vi "Stepper motor B.vi"(6 "Microstep size":T1(ring), 7 "Speed":u32=5, 8 "error in (no error)":errorcluster, 9 "Direction (A/DIO5 (Pin 21))":bool, 10 "Step (A/DIO4 (Pin 19))":bool, 11 "Enable (A/DIO0 (Pin 11))":bool) -> (0 "error out":errorcluster, 2 "Direction":bool)   [LabVIEW 2015]
uses:
  <vilib>/myRIO/Instrument Drivers/Onboard IO/DIO/DIO.lvlib
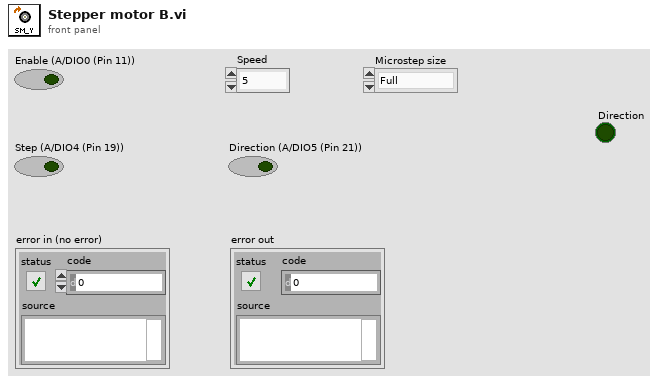
[diagram p1: front panel]
types:
  T1 = enum16{"Full", "Half", "Quarter", "Eighth", "Sixteenth"}
  T2 = cluster{"MS1 (A/DIO1 (Pin 13))":bool, "MS2 (A/DIO2 (Pin 15))":bool, "MS3 (A/DIO3 (Pin 17))":bool}
  T3 = typedef "DIO.lvlib/DIO Reference.ctl" = cluster{"myRIO Reference":T4, "DIO Channels List":T8}
  T4 = typedef "myRIO Generic Hardware Reference.ctl" = cluster{"myRIO Model":T5, "myRIO Hardware Reference":T6}
  T5 = typedef "Hardware Version Enum.ctl" = enum16{"Unknown", "myRIO-1900", "myRIO-1950", "roboRIO", "NI ELVIS RIO CM"}
  T6 = typedef "myRIO v1.0 Reference.ctl" = cluster{"Generic FPGA Reference":T7, "Allow multiple opens":bool}
  T7 = typedef "Generic FPGA Reference.ctl" = refnum<k20>
  T8 = typedef "DIO Channels List.ctl" = T9[]
  T9 = typedef "DIO Channels Enum.ctl" = enum16{"Not Connected", "C/DIO0", "C/DIO1", "C/DIO2", "C/DIO3", "C/DIO4", "C/DIO5", "C/DIO6", "C/DIO7", "A/DIO0", "A/DIO1", "A/DIO2", "A/DIO3", "A/DIO4", "A/DIO5", "A/DIO6", "A/DIO7", "A/DIO8", "A/DIO9", "A/DIO10", "A/DIO11", "A/DIO12", "A/DIO13", "A/DIO14", "A/DIO15", "B/DIO0", "B/DIO1", "B/DIO2", "B/DIO3", "B/DIO4", "B/DIO5", "B/DIO6", "B/DIO7", "B/DIO8", "B/DIO9", "B/DIO10", "B/DIO11", "B/DIO12", "B/DIO13", "B/DIO14", "B/DIO15", "LED0", "LED1", "LED2", "LED3", "Button0", "DIO/DIO0", "DIO/DIO1", "DIO/DIO2", "DIO/DIO3", "DIO/DIO4", "DIO/DIO5", "DIO/DIO6", "DIO/DIO7", "DIO/DIO8", "DIO/DIO9", "SPI/CS0", "SPI/CS1", "SPI/CS2", "SPI/CS3", "LED RADIO (Green)", "LED RADIO (Red)", "LED COMM (Green)", "LED COMM (Red)", "LED MODE (Green)", "LED MODE (Red)"}
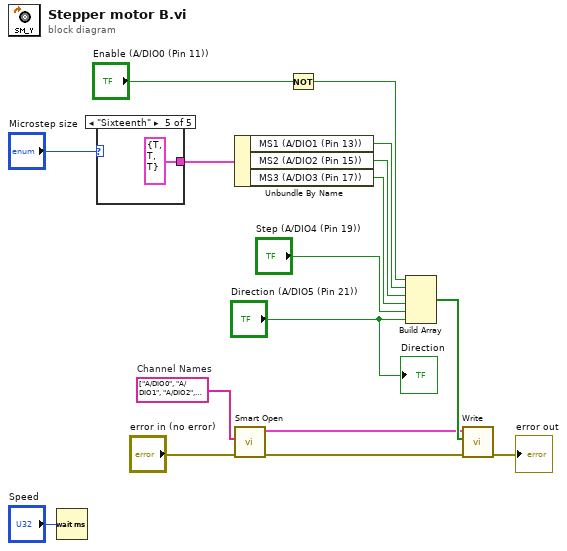
[diagram p0: block diagram]
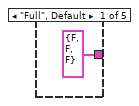
[diagram p2: hidden frame]
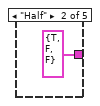
[diagram p3: hidden frame]
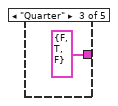
[diagram p4: hidden frame]
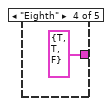
[diagram p5: hidden frame]
diagram:
  w14 = tag[] ["A/DIO0", "A/DIO1", "A/DIO2", "A/DIO3", "A/DIO4", "A/DIO5"]  # Channel Names
  n1 = Wait (ms)(milliseconds to wait="Speed") -> ()  [unwired: 1 out]
  n2 = case shown="\"Sixteenth\"" "Microstep size" {
    tunnel: [T2 {"MS1 (A/DIO1 (Pin 13))"=FALSE, "MS2 (A/DIO2 (Pin 15))"=FALSE, "MS3 (A/DIO3 (Pin 17))"=FALSE} ("Microstepping") T2 {"MS1 (A/DIO1 (Pin 13))"=TRUE, "MS2 (A/DIO2 (Pin 15))"=FALSE, "MS3 (A/DIO3 (Pin 17))"=FALSE} ("Microstepping") T2 {"MS1 (A/DIO1 (Pin 13))"=FALSE, "MS2 (A/DIO2 (Pin 15))"=TRUE, "MS3 (A/DIO3 (Pin 17))"=FALSE} ("Microstepping") T2 {"MS1 (A/DIO1 (Pin 13))"=TRUE, "MS2 (A/DIO2 (Pin 15))"=TRUE, "MS3 (A/DIO3 (Pin 17))"=FALSE} ("Microstepping") T2 {"MS1 (A/DIO1 (Pin 13))"=TRUE, "MS2 (A/DIO2 (Pin 15))"=TRUE, "MS3 (A/DIO3 (Pin 17))"=TRUE} ("Microstepping")] -> w1
    frame "Full", Default {
    }
    frame "Half" {
    }
    frame "Quarter" {
    }
    frame "Eighth" {
    }
    frame "Sixteenth" {
    }
  }
  n3 = Unbundle By Name(w1) -> ("MS1 (A/DIO1 (Pin 13))"=w9:bool, "MS2 (A/DIO2 (Pin 15))"=w8:bool, "MS3 (A/DIO3 (Pin 17))"=w7:bool)
  n4 = call <vilib>:"Smart Open.vi"("error in (no error)"="error in (no error)", "Channel Names"=w14) -> ("error out"=w11:errorcluster, "DIO Ref Out"=w12:T3)  [unwired: 8 in]
  n5 = Not(x="Enable (A/DIO0 (Pin 11))") -> (.not. x?=w10:bool)
  n6 = Build Array(w10, w9, w8, w7, "Step (A/DIO4 (Pin 19))", "Direction (A/DIO5 (Pin 21))") -> (w13:bool[])
  n7 = call <vilib>:"Write.vi"("error in (no error)"=w11, "Values"=w13, "DIO Ref In"=w12) -> ("error out"=→"error out":errorcluster)  [unwired: 6 in, 1 out]
  "Direction" <- "Direction (A/DIO5 (Pin 21))"
